vi "Set Tuner Gain.vi"(8 "error in (no error)":errorcluster, 10 "Gain (dB)":dbl, 11 "DeviceRefnum":u64) -> (0 "error out":errorcluster, 2 "function return":i32, 3 "DeviceRefnum Out":u64)   [LabVIEW 2016]
doc: "RTLSDR_API int rtlsdr_set_tuner_gain(rtlsdr_dev_t *dev, int gain);"
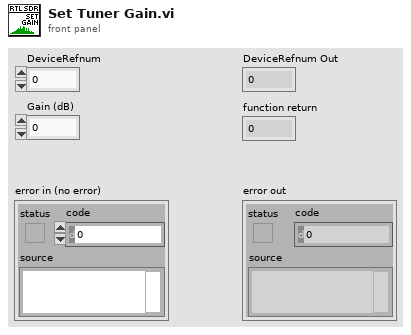
[diagram p1: front panel]
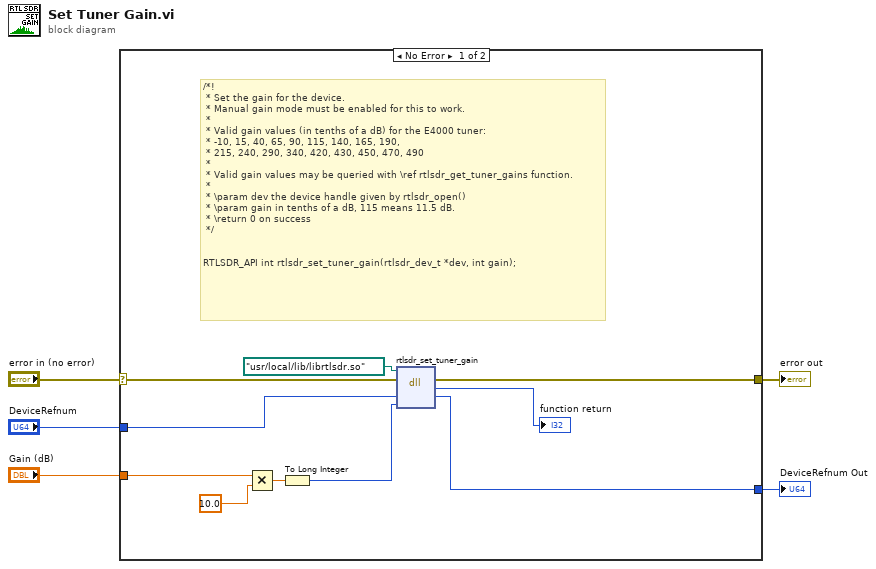
[diagram p0: block diagram]
diagram:
  n1 = case shown="No Error" "error in (no error)" {
    selector: "error in (no error)" -> [w8 w17]
    tunnel: [w14 w17] -> w5
    tunnel: "Gain (dB)" -> [w13 _]
    tunnel: "DeviceRefnum" -> [w9 w16]
    tunnel: [w6 w16] -> w1
    frame No Error {
      # "/*!\n * Set the gain for the device.\n * Manual gain mode must be enabled for this to work.\n *\n * Valid gain values (in tenths of a dB) for the E4000 tuner:\n * -10, 15, 40, 65, 90, 115, 140, 165, 190,\n * 215, 240, 290, 340, 420, 430, 450, 470, 490\n *\n * Valid gain values may be queried with \\ref rtlsdr_get_tuner_gains function.\n *\n * \\param dev the device handle given by rtlsdr_open()\n * \\param gain in tenths of a dB, 115 means 11.5 dB.\n * \\return 0 on success\n */\n\n\nRTLSDR_API int rtlsdr_set_tuner_gain(rtlsdr_dev_t *dev, int gain);"
      n2 = Multiply(x=w13, y=10.0) -> (x*y=w11:dbl)
      n3 = To Long Integer(number=w11) -> (32bit integer=w10:i32)
      n4 = dll-call lib="C:/Program Files (x86)/National Instruments/LabVIEW 2016/user.lib/rtlsdr/rtlsdr.*" fn="rtlsdr_set_tuner_gain"(path in=path "/usr/local/lib/librtlsdr.so", error in=w8, "DeviceRefnum"=w9, "Gain"=w10) -> (error out=w14:errorcluster, "return type"=→"function return":i32, "DeviceRefnum"=w6:u64)  [unwired: 2 in, 1 out]
    }
    frame Error {
    }
  }
  "error out" <- w5
  "DeviceRefnum Out" <- w1
